vi "Start Panel Array.vi"(8 "error in (no error)":errorcluster, 11 "GVIWebProcessorApp in":refnum<class "GVIWebProcessorApp.lvclass">) -> (0 "error out":errorcluster, 3 "GVIWebProcessorApp out":refnum<class "GVIWebProcessorApp.lvclass">)   [LabVIEW 2020, in "PicoG-Processor.lvlib" / "GVIWebProcessorApp.lvclass"]
uses:
  GVIWebProcessorApp.lvclass
  <vilib>/IlluminatedG/IG OOPanel/OOPanel/ArrayManager/ArrayManager.lvclass
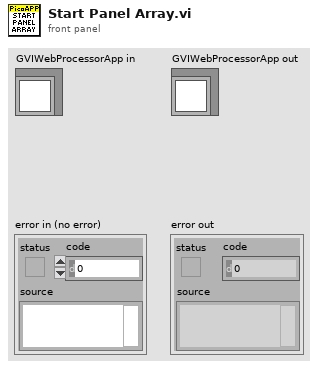
[diagram p1: front panel]
types:
  T1 = typedef "PicoG-Processor.lvlib/GVIWebProcessorApp.lvclass/UI Refs.ctl" = cluster{"Main Window":refnum<vi>, "List Panel":refnum<vi>, "H Splitter":refnum<vi>, "V Splitter":refnum<vi>, "Open Project":refnum<vi>, "Project Name":refnum<vi>, "Auto Process":refnum<vi>, "Auto Deploy":refnum<vi>, "Process Platform":refnum<vi>, "Last Target":refnum<vi>}
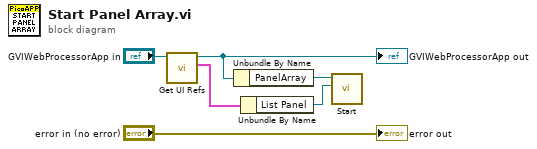
[diagram p0: block diagram]
diagram:
  n1 = call "Get UI Refs.vi"("GVIWebProcessorApp in"="GVIWebProcessorApp in") -> ("UI Refs"=w2:T1, "GVIWebProcessorApp out"=w3:refnum<class "GVIWebProcessorApp.lvclass">)  [unwired: 8 in, 1 out]
  "GVIWebProcessorApp out" <- w3
  n2 = Unbundle By Name(w3) -> ("PanelArray"=w5:refnum<class "ArrayManager.lvclass">)
  n3 = Unbundle By Name(w2) -> ("List Panel"=w1:refnum<vi>)
  n4 = call <vilib>:"Start.vi"("Container"=w1, "ArrayManager in"=w5) -> ()  [unwired: 8 in, 2 out]
  "error out" <- "error in (no error)"
